vi "cs_combinePseudoGellerman.vi"(8 "error in (no error)":errorcluster, 10 "Input2":dbl[][](array[numeric]), 11 "Input1":dbl[][](array[numeric])) -> (0 "error out":errorcluster, 3 "Output":dbl[][](array[numeric]))   [LabVIEW 2013]
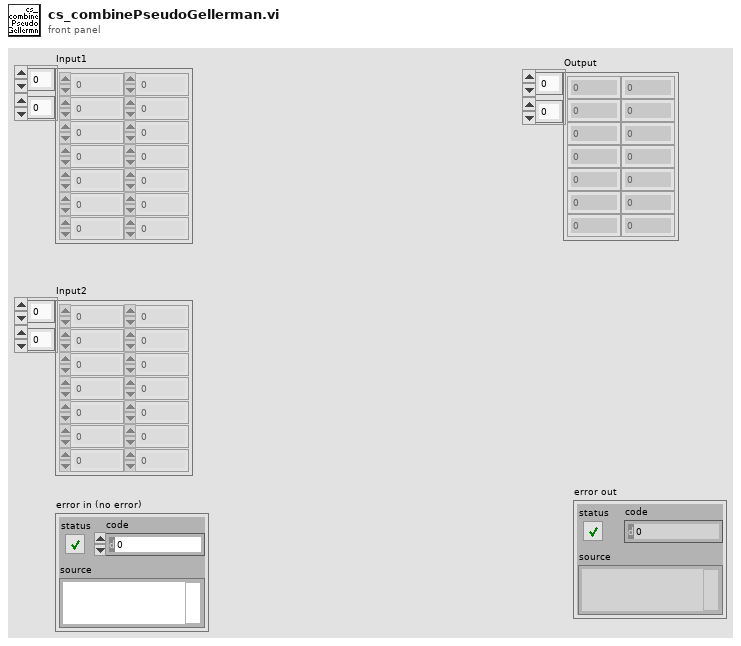
[diagram p1: front panel]
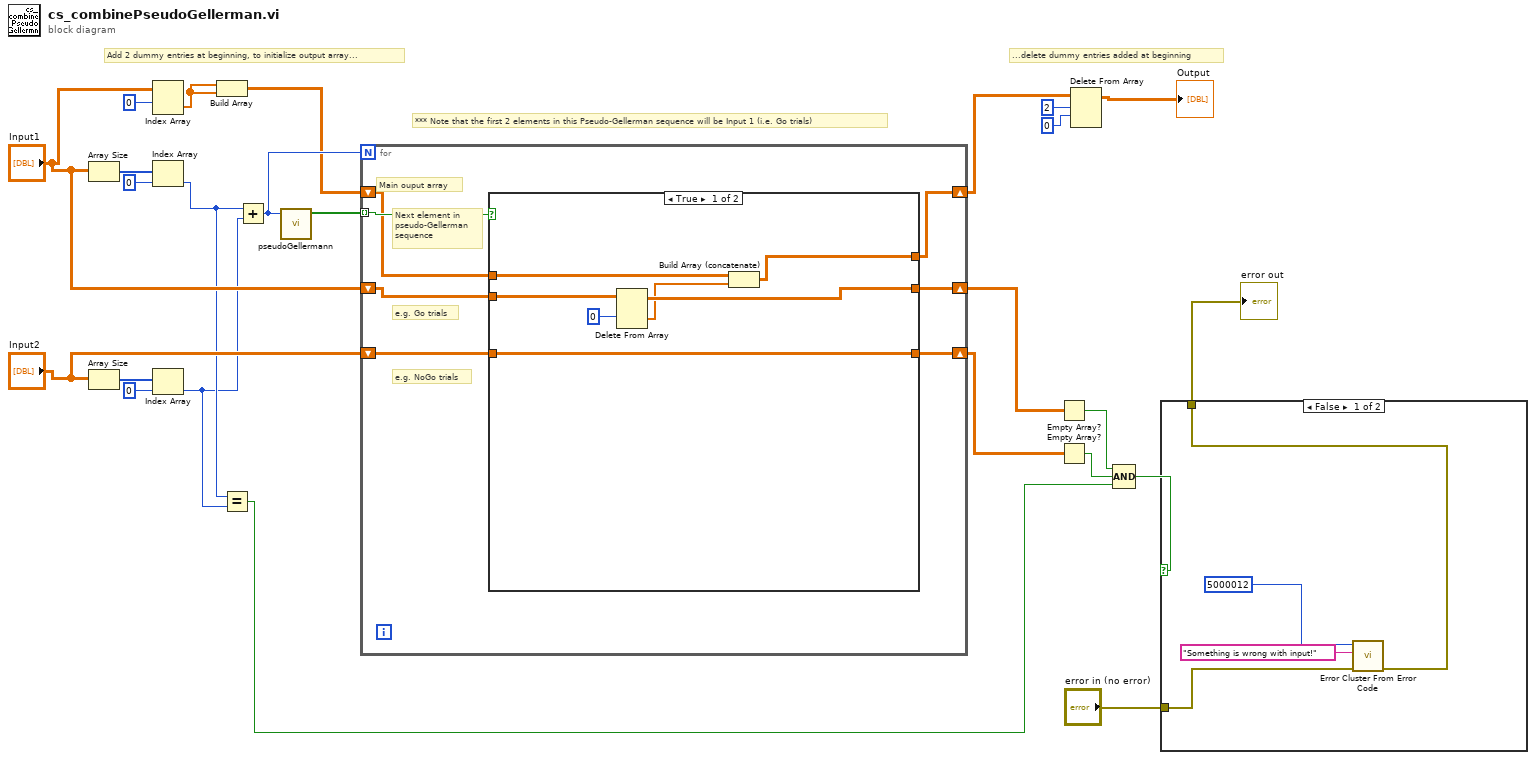
[diagram p0: block diagram]
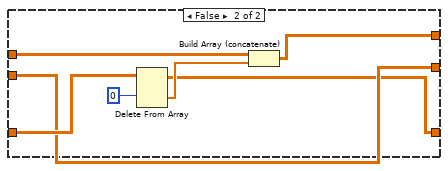
[diagram p3: hidden frame]
diagram:
  # "*** Note that the first 2 elements in this Pseudo-Gellerman sequence will be Input 1 (i.e. Go trials)"
  # "Add 2 dummy entries at beginning, to initialize output array..."
  # "...delete dummy entries added at beginning"
  n1 = Array Size(array="Input1") -> (size(s)=w25:i32[])
  n2 = Array Size(array="Input2") -> (size(s)=w23:i32[])
  n3 = Index Array(array="Input1", index (row)=0) -> (element=w16:dbl[])  [unwired: 1 in]
  n4 = Index Array(array=w25, index=0) -> (element=w10:i32)
  n5 = Index Array(array=w23, index=0) -> (element=w9:i32)
  n6 = Build Array(w16, w16) -> (w15:dbl[][])
  n7 = Equal?(x=w10, y=w9) -> (x = y?=w4:bool)
  n8 = Add(x=w10, y=w9) -> (x+y=w21:i32)
  n9 = call "pseudoGellermann.vi"("N"=w21) -> ("Array"=w20:bool[])  [unwired: 10 in]
  n10 = for {
    N: w21 -> [_]
    tunnel: w20 -> [w32] mode=indexing
    shift-right: [w26] -> w14
    shift-left: w15 -> [w31]
    shift-right: [w29] -> w8
    shift-left: "Input1" -> [w30]
    shift-right: [w27] -> w7
    shift-left: "Input2" -> [w28]
    # "e.g. NoGo trials"
    # "e.g. Go trials"
    # "Next element in\npseudo-Gellerman\nsequence"
    # "Main ouput array"
    n11 = case shown="True" w32 {
      tunnel: w31 -> [w39 w46]
      tunnel: w30 -> [w38 w41]
      tunnel: [w37 w41] -> w29
      tunnel: w28 -> [w34 w42]
      tunnel: [w34 w40] -> w27
      tunnel: [w33 w44] -> w26
      frame True {
        n12 = Delete From Array(array=w38, index (row)=0) -> (deleted portion=w36:dbl[], array with subset deleted=w37:dbl[][])  [unwired: 2 in]
        n13 = Build Array (concatenate)(w39, w36) -> (w33:dbl[][])
      }
      frame False {
        n14 = Delete From Array(array=w42, index (row)=0) -> (deleted portion=w43:dbl[], array with subset deleted=w40:dbl[][])  [unwired: 2 in]
        n15 = Build Array (concatenate)(w46, w43) -> (w44:dbl[][])
      }
    }
  }
  n16 = Empty Array?(array=w8) -> (empty?=w6:bool)
  n17 = Empty Array?(array=w7) -> (empty?=w5:bool)
  n18 = Delete From Array(array=w14, length=2, index (row)=0) -> (array with subset deleted=→"Output":dbl[][])  [unwired: 1 in, 1 out]
  n19 = Compound Arithmetic op=AND(w6, w5, w4) -> (w3:bool)
  n20 = case shown="False" w3 {
    tunnel: "error in (no error)" -> [w50 w51]
    tunnel: [w49 w51] -> w1
    frame False {
      n21 = call <vilib>:"Error Cluster From Error Code.vi"("error in (no error)"=w50, "error message (\"\")"="Something is wrong with input!" ("error message (\"\")"), "error code (0)"=5000012) -> ("error out"=w49:errorcluster)  [unwired: 6 in]
    }
    frame True {
    }
  }
  "error out" <- w1
